vi "startUp.vi"(8 "error in (no error)":errorcluster, 10 "HardwareList out":refnum<class "HWConfiguration.lvclass">, 11 "AtomChipHWC in":refnum<class "AtomChipHWC.lvclass">) -> (0 "error out":errorcluster, 3 "AtomChipHWC out":refnum<class "AtomChipHWC.lvclass">)   [LabVIEW 2009, in "Hardware.lvlib" / "HWControllers.lvlib" / "AtomChipHWC.lvclass"]
doc: "Opens the devices ready for use."
uses:
  AtomChipHWC.lvclass
  HardwareConfiguration/HWConfiguration.lvclass
  AtomChipHWC.lvclass/AtomChipHWC.ctl
  Channels/Digital/DigitalOutput.lvclass
  Channels/VoltOutput/AnalogOutput.lvclass
  HWController.lvclass
  Channels/DDSOutput/Generic/DDSOutput.lvclass
  Network Controllers/CameraNetworkController/CameraNetworkController.lvclass
  Network Controllers/NetworkCamera/NetworkCamera.lvclass
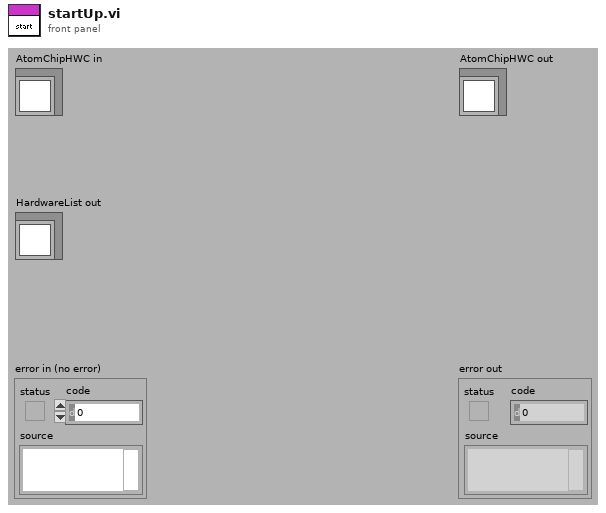
[diagram p1: front panel]
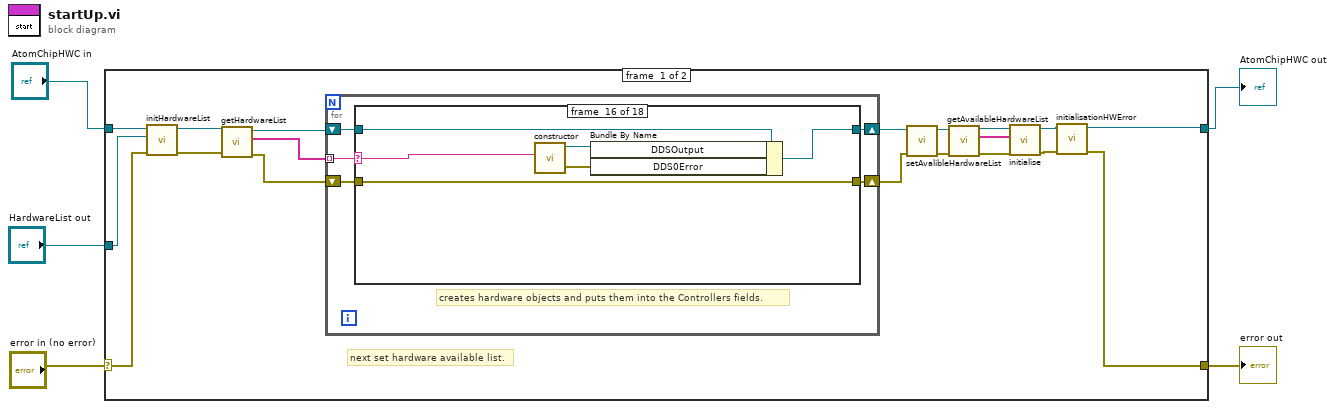
[diagram p0: block diagram]
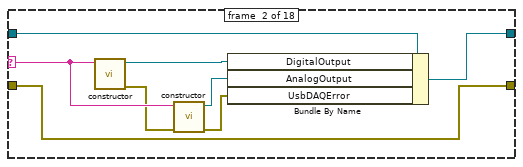
[diagram p3: hidden frame]
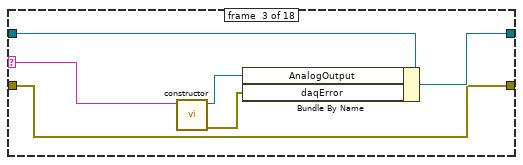
[diagram p4: hidden frame]
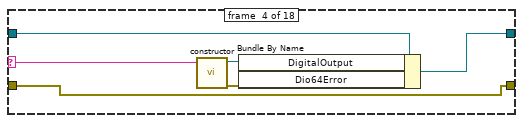
[diagram p5: hidden frame]
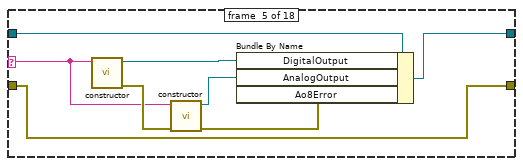
[diagram p6: hidden frame]
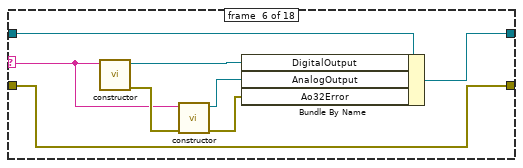
[diagram p7: hidden frame]
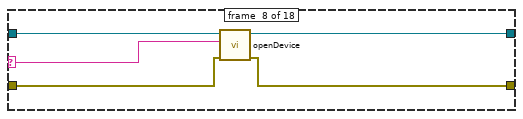
[diagram p9: hidden frame]
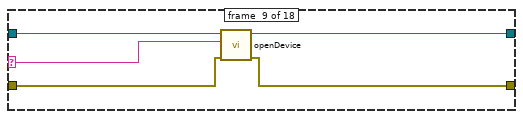
[diagram p10: hidden frame]
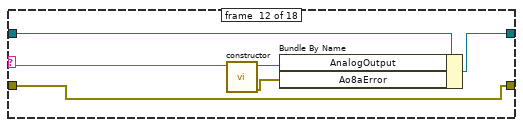
[diagram p13: hidden frame]
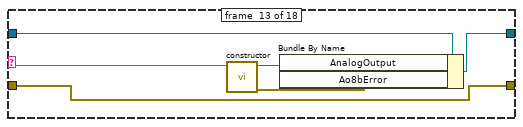
[diagram p14: hidden frame]
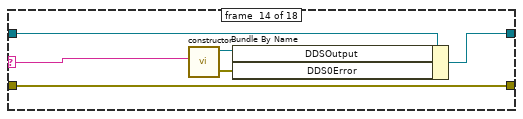
[diagram p15: hidden frame]
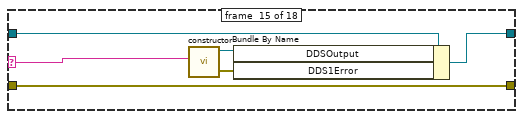
[diagram p16: hidden frame]
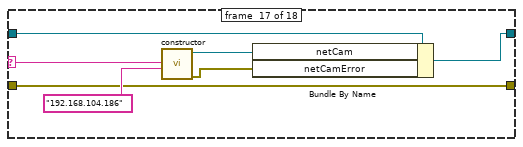
[diagram p17: hidden frame]
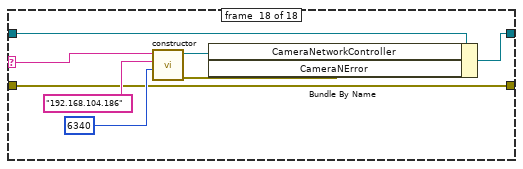
[diagram p18: hidden frame]
diagram:
  n1 = case shown="No Error" "error in (no error)" {
    selector: "error in (no error)" -> [w11 w129]
    tunnel: [w6 w129] -> w4
    tunnel: "AtomChipHWC in" -> [w12 w130]
    tunnel: [w7 w130] -> w2
    tunnel: "HardwareList out" -> [w10 _]
    frame #0 {
      # "next set hardware available list."
      n2 = call-dynamic "initHardwareList.vi"("error in (no error)"=w11, "HardwareList out"=w10, "AtomChipHWC in"=w12) -> ("error out"=w20:errorcluster, "AtomChipHWC out"=w22:refnum<class "AtomChipHWC.lvclass">)  [unwired: 7 in]
      n3 = call "getHardwareList.vi"("error in (no error)"=w20, "HWController.lvclass in"=w22) -> ("error out"=w19:errorcluster, "HardwareList"=w18:string[], "HWController.lvclass out"=w21:refnum<class "AtomChipHWC.lvclass">)  [unwired: 7 in]
      n4 = for {
        tunnel: w18 -> [w25] mode=indexing
        shift-right: [w28] -> w24
        shift-left: w21 -> [w29]
        shift-right: [w26] -> w23
        shift-left: w19 -> [w27]
        # "creates hardware objects and puts them into the Controllers fields."
        n5 = case shown="\"Pixelfly\", \"ProEM_WinX32\"" w25 {
          selector: w25 -> [_ w39 w42 w48 w56 w62 _ w70 w75 _ _ w86 w92 w98 w104 w110 w116 w128]
          tunnel: w29 -> [w31 w37 w44 w49 w55 w64 w69 w74 w79 w81 w83 w89 w95 w101 w107 w113 w120 w125]
          tunnel: [w31 w34 w43 w50 w54 w63 w69 w73 w78 w81 w83 w88 w94 w100 w106 w112 w119 w124] -> w28
          tunnel: w27 -> [w30 w32 w40 w46 w52 w60 w68 w72 w76 w80 w82 w84 w90 w96 w102 w108 w114 w121]
          tunnel: [w30 w32 w40 w46 w52 w60 w68 w71 w77 w80 w82 w84 w90 w96 w102 w108 w114 w121] -> w26
          frame #0 {
          }
          frame #1 {
            n6 = call "constructor.vi"("deviceName"=w39) -> ("error out"=w38:errorcluster, "DigitalOutput out"=w36:refnum<class "DigitalOutput.lvclass">)  [unwired: 9 in]
            n7 = call "constructor.vi"("error in (no error)"=w38, "deviceName"=w39) -> ("error out"=w33:errorcluster, "AnalogOutput out"=w35:refnum<class "AnalogOutput.lvclass">)  [unwired: 8 in]
            n8 = Bundle By Name(cluster=w37, "DigitalOutput"=w36, "AnalogOutput"=w35, "UsbDAQError"=w33) -> (w34:refnum<class "AtomChipHWC.lvclass">)
          }
          frame #2 {
            n9 = call "constructor.vi"("deviceName"=w42) -> ("error out"=w41:errorcluster, "AnalogOutput out"=w45:refnum<class "AnalogOutput.lvclass">)  [unwired: 9 in]
            n10 = Bundle By Name(cluster=w44, "AnalogOutput"=w45, "daqError"=w41) -> (w43:refnum<class "AtomChipHWC.lvclass">)
          }
          frame #3 {
            n11 = call "constructor.vi"("deviceName"=w48) -> ("error out"=w47:errorcluster, "DigitalOutput out"=w51:refnum<class "DigitalOutput.lvclass">)  [unwired: 9 in]
            n12 = Bundle By Name(cluster=w49, "DigitalOutput"=w51, "Dio64Error"=w47) -> (w50:refnum<class "AtomChipHWC.lvclass">)
          }
          frame #4 {
            n13 = call "constructor.vi"("deviceName"=w56) -> ("error out"=w59:errorcluster, "DigitalOutput out"=w58:refnum<class "DigitalOutput.lvclass">)  [unwired: 9 in]
            n14 = call "constructor.vi"("error in (no error)"=w59, "deviceName"=w56) -> ("error out"=w53:errorcluster, "AnalogOutput out"=w57:refnum<class "AnalogOutput.lvclass">)  [unwired: 8 in]
            n15 = Bundle By Name(cluster=w55, "DigitalOutput"=w58, "AnalogOutput"=w57, "Ao8Error"=w53) -> (w54:refnum<class "AtomChipHWC.lvclass">)
          }
          frame #5 {
            n16 = call "constructor.vi"("deviceName"=w62) -> ("error out"=w67:errorcluster, "DigitalOutput out"=w66:refnum<class "DigitalOutput.lvclass">)  [unwired: 9 in]
            n17 = call "constructor.vi"("error in (no error)"=w67, "deviceName"=w62) -> ("error out"=w61:errorcluster, "AnalogOutput out"=w65:refnum<class "AnalogOutput.lvclass">)  [unwired: 8 in]
            n18 = Bundle By Name(cluster=w64, "DigitalOutput"=w66, "AnalogOutput"=w65, "Ao32Error"=w61) -> (w63:refnum<class "AtomChipHWC.lvclass">)
          }
          frame #6 {
          }
          frame #7 {
            n19 = call "openDevice.vi"("error in (no error)"=w72, "deviceName"=w70, "AtomChipHWC in"=w74) -> ("error out"=w71:errorcluster, "AtomChipHWC out"=w73:refnum<class "AtomChipHWC.lvclass">)  [unwired: 7 in]
          }
          frame #8 {
            n20 = call "openDevice.vi"("error in (no error)"=w76, "deviceName"=w75, "AtomChipHWC in"=w79) -> ("error out"=w77:errorcluster, "AtomChipHWC out"=w78:refnum<class "AtomChipHWC.lvclass">)  [unwired: 7 in]
          }
          frame #9 {
          }
          frame #10 {
          }
          frame #11 {
            n21 = call "constructor.vi"("deviceName"=w86) -> ("error out"=w85:errorcluster, "AnalogOutput out"=w87:refnum<class "AnalogOutput.lvclass">)  [unwired: 9 in]
            n22 = Bundle By Name(cluster=w89, "AnalogOutput"=w87, "Ao8aError"=w85) -> (w88:refnum<class "AtomChipHWC.lvclass">)
          }
          frame #12 {
            n23 = call "constructor.vi"("deviceName"=w92) -> ("error out"=w91:errorcluster, "AnalogOutput out"=w93:refnum<class "AnalogOutput.lvclass">)  [unwired: 9 in]
            n24 = Bundle By Name(cluster=w95, "AnalogOutput"=w93, "Ao8bError"=w91) -> (w94:refnum<class "AtomChipHWC.lvclass">)
          }
          frame #13 {
            n25 = call "constructor.vi"("device"=w98) -> ("error out"=w97:errorcluster, "DDSOutput out"=w99:refnum<class "DDSOutput.lvclass">)  [unwired: 9 in]
            n26 = Bundle By Name(cluster=w101, "DDSOutput"=w99, "DDS0Error"=w97) -> (w100:refnum<class "AtomChipHWC.lvclass">)
          }
          frame #14 {
            n27 = call "constructor.vi"("device"=w104) -> ("error out"=w103:errorcluster, "DDSOutput out"=w105:refnum<class "DDSOutput.lvclass">)  [unwired: 9 in]
            n28 = Bundle By Name(cluster=w107, "DDSOutput"=w105, "DDS1Error"=w103) -> (w106:refnum<class "AtomChipHWC.lvclass">)
          }
          frame #15 {
            n29 = call "constructor.vi"("device"=w110) -> ("error out"=w109:errorcluster, "DDSOutput out"=w111:refnum<class "DDSOutput.lvclass">)  [unwired: 9 in]
            n30 = Bundle By Name(cluster=w113, "DDSOutput"=w111, "DDS0Error"=w109) -> (w112:refnum<class "AtomChipHWC.lvclass">)
          }
          frame #16 {
            n31 = call "constructor.vi"("machine name"="192.168.104.186" ("remote address"), "Camera"=w116) -> ("error out"=w117:errorcluster, "NetworkCamera out"=w118:refnum<class "NetworkCamera.lvclass">)  [unwired: 8 in]
            n32 = Bundle By Name(cluster=w120, "netCam"=w118, "netCamError"=w117) -> (w119:refnum<class "AtomChipHWC.lvclass">)
          }
          frame #17 {
            n33 = call "constructor.vi"("remote port"=u16 6340, "remote address"="192.168.104.186", "camera"=w128) -> ("error out"=w122:errorcluster, "CameraNetworkController out"=w123:refnum<class "CameraNetworkController.lvclass">)  [unwired: 7 in]
            n34 = Bundle By Name(cluster=w125, "CameraNetworkController"=w123, "CameraNError"=w122) -> (w124:refnum<class "AtomChipHWC.lvclass">)
          }
        }
      }
      n35 = call "setAvalibleHardwareList.vi"("error in (no error)"=w23, "HWController in"=w24) -> ("error out"=w16:errorcluster, "HWController out"=w17:refnum<class "AtomChipHWC.lvclass">)  [unwired: 8 in]
      n36 = call "getAvailableHardwareList.vi"("error in (no error)"=w16, "HWController.lvclass in"=w17) -> ("error out"=w14:errorcluster, "AvailableHardwareList"=w13:string[], "HWController.lvclass out"=w15:refnum<class "AtomChipHWC.lvclass">)  [unwired: 7 in]
      n37 = call-dynamic "initialise.vi"("error in (no error)"=w14, "HWList"=w13, "AtomChipHWC in"=w15) -> ("error out"=w8:errorcluster, "AtomChipHWC out"=w9:refnum<class "AtomChipHWC.lvclass">)  [unwired: 7 in]
      n38 = call-dynamic "initialisationHWError.vi"("error in (no error)"=w8, "AtomChipHWC in"=w9) -> ("error out"=w6:errorcluster, "AtomChipHWC out"=w7:refnum<class "AtomChipHWC.lvclass">)  [unwired: 8 in]
    }
    frame #1 {
    }
  }
  "error out" <- w4
  "AtomChipHWC out" <- w2
